vi "Get Last Temperature.vi"(8 "error in":errorcluster, 10 "Channel":string, 11 "Thermometer DAQmx RTD Cont CFG in":refnum<class "Thermometer DAQmx RTD Cont CFG.lvclass">) -> (0 "error out":errorcluster, 2 "Temperature":dbl, 3 "Thermometer DAQmx RTD Cont CFG out":refnum<class "Thermometer DAQmx RTD Cont CFG.lvclass">)   [LabVIEW 2023, in "Thermometer DAQmx RTD Cont CFG.lvclass"]
uses:
  Thermometer DAQmx RTD Cont CFG.lvclass
  Thermometer DAQmx RTD Cont CFG.lvclass/Thermometer DAQmx RTD Cont CFG.ctl
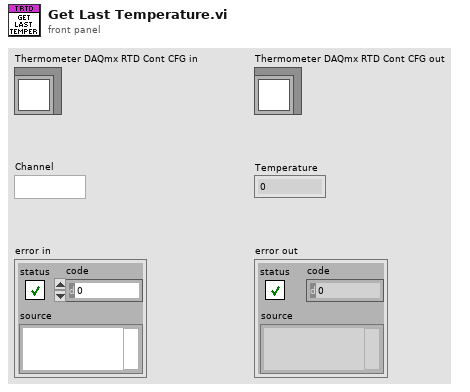
[diagram p1: front panel]
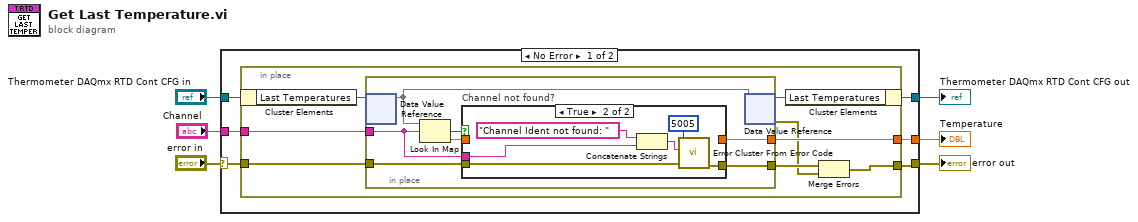
[diagram p0: block diagram]
diagram:
  n1 = case shown="No Error" "error in" {
    selector: "error in" -> [w10 w37]
    tunnel: [w9 w37] -> w5
    tunnel: [w7 w36] -> w3
    tunnel: "Thermometer DAQmx RTD Cont CFG in" -> [w12 w36]
    tunnel: "Channel" -> [w11 _]
    tunnel: [w8 _] -> w1
    frame No Error {
      n2 = in-place {
        in-place-border: w11 -> [w19]
        in-place-border: w10 -> [w18]
        in-place-border: [w14] -> w9
        in-place-border: [w16] -> w8
        n3 = in-place-cluster #1(w12) -> ("Last Temperatures"=w20:refnum<data-value>)
        n4 = in-place {
          in-place-border: w19 -> [w25]
          in-place-border: w18 -> [w26]
          in-place-border: [w24] -> w17
          in-place-border: [w22] -> w16
          n5 = in-place-dvr #2(w20) -> (w21:map{string, dbl})  [unwired: 1 out]
          n6 = Look In Map(map=w21, key=w25) -> (key not found?=w27:bool, value=w23:dbl)  [unwired: 1 in]
          n7 = case "Channel not found?" shown="True" w27 {
            tunnel: w26 -> [w29 w35]
            tunnel: w25 -> [_ w31]
            tunnel: [w29 w30] -> w24
            tunnel: w23 -> [w28 _]
            tunnel: [w28 _] -> w22
            frame False {
            }
            frame True {
              n8 = Concatenate Strings("Channel Ident not found: " ("error message (\"\")"), w31) -> (w33:string)
              n9 = call <vilib>:"Error Cluster From Error Code.vi"("error in (no error)"=w35, "error message (\"\")"=w33, "error code (0)"=5005) -> ("error out"=w30:errorcluster)  [unwired: 6 in]
            }
          }
          n10 = in-place-dvr #2(w21) -> (w15:refnum<data-value>, w13:errorcluster)
        }
        n11 = in-place-cluster #1("Last Temperatures"=w15) -> (w7:refnum<class "Thermometer DAQmx RTD Cont CFG.lvclass">)
        n12 = Merge Errors(w17, w13) -> (w14:errorcluster)
      }
    }
    frame Error {
    }
  }
  "error out" <- w5
  "Thermometer DAQmx RTD Cont CFG out" <- w3
  "Temperature" <- w1
